vi "Register For Events.vi"(8 "error in (no error)":errorcluster, 11 "TwinCAT ADS in":refnum<class "TwinCAT ADS.lvclass">) -> (0 "error out":errorcluster, 2 "Event Registration Refnum":refnum<event-registration>, 3 "TwinCAT ADS out":refnum<class "TwinCAT ADS.lvclass">)   [LabVIEW 2018, in "TwinCAT ADS.lvclass"]
uses:
  TwinCAT ADS.lvclass
  Controls/ADS Notification Event Data.ctl
  Controls/Symbol Information.ctl
  Controls/State Information.ctl
  Controls/Connection State Change Event Data.ctl
  Controls/AMS Router Notification Event Data.ctl
  Controls/AMS Router State.ctl
  TwinCAT ADS.lvclass/TwinCAT ADS.ctl
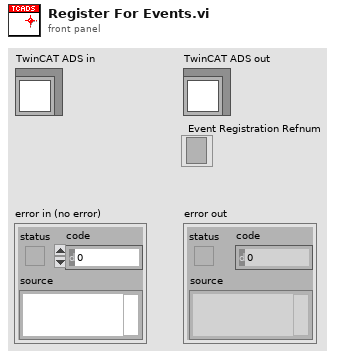
[diagram p1: front panel]
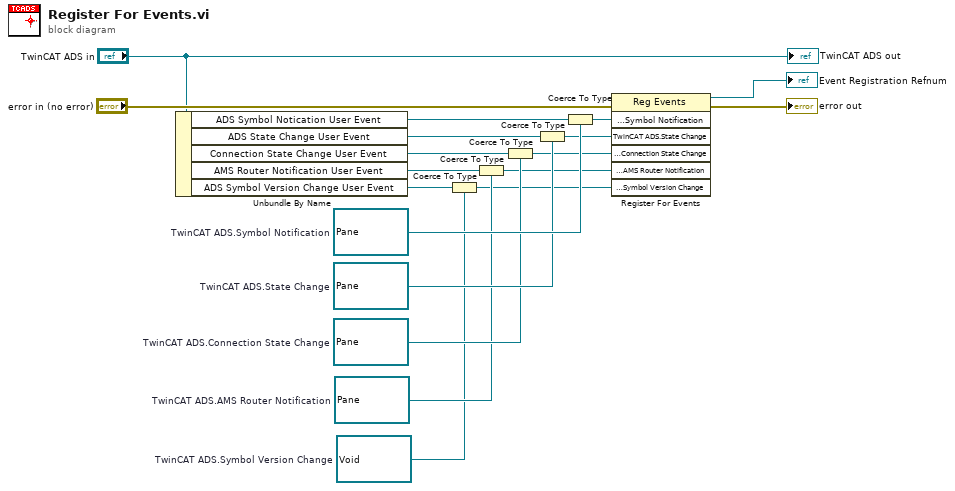
[diagram p0: block diagram]
diagram:
  w8 = refnum<user-event> refnum  # TwinCAT ADS.AMS Router Notification
  w7 = refnum<user-event> refnum  # TwinCAT ADS.Symbol Version Change
  w9 = refnum<user-event> refnum  # TwinCAT ADS.Connection State Change
  w10 = refnum<user-event> refnum  # TwinCAT ADS.State Change
  w11 = refnum<user-event> refnum  # TwinCAT ADS.Symbol Notification
  n1 = Unbundle By Name("TwinCAT ADS in") -> ("ADS Symbol Notication User Event"=w16:refnum<user-event>, "ADS State Change User Event"=w15:refnum<user-event>, "Connection State Change User Event"=w14:refnum<user-event>, "AMS Router Notification User Event"=w13:refnum<user-event>, "ADS Symbol Version Change User Event"=w12:refnum<user-event>)
  n2 = Coerce To Type(0:w12, 1:w7) -> (2:w2:refnum<user-event>)
  n3 = Coerce To Type(0:w13, 1:w8) -> (2:w3:refnum<user-event>)
  n4 = Coerce To Type(0:w14, 1:w9) -> (2:w4:refnum<user-event>)
  n5 = Coerce To Type(0:w15, 1:w10) -> (2:w5:refnum<user-event>)
  n6 = Coerce To Type(0:w16, 1:w11) -> (2:w6:refnum<user-event>)
  n7 = register-events(error in="error in (no error)", w6, w5, w4, w3, w2) -> (reference out=→"Event Registration Refnum":refnum<event-registration>, error out=→"error out":errorcluster)  [unwired: 1 in]
  "TwinCAT ADS out" <- "TwinCAT ADS in"
